vi "PicoScope6000GetTriggerInfo.vi"(0 "handle in":i16, 5 "Segment Range":T1={"fromSegmentIndex"=0, "toSegmentIndex"=9} {"toSegmentIndex" format="%.4p"; "fromSegmentIndex" format="%.4p"}, 9 "Sample Rate":sgl, 11 "error in":errorcluster) -> (4 "handle out":i16, 6 "Trigger Info":T2(array[cluster]), 10 "Trigger Offsets":cluster{u64, sgl}[](array[cluster]) {"?" format="%#_5p"}, 15 "error out":errorcluster)   [LabVIEW 2010]
doc: "This VI gets trigger timestamped data using rapid block mode. It outputs one-dimensional array for each memory segment."
uses:
  ps6000.dll
  shared/Segment Range.ctl
panel:
  out "Number of Captures":u32=1
  in  "fromSegmentIndex":u32
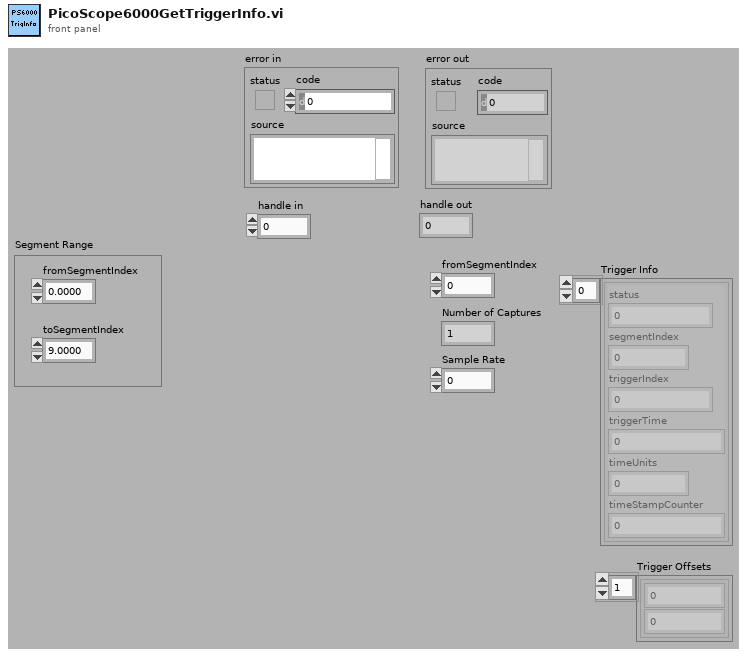
[diagram p1: front panel]
types:
  T1 = typedef "Segment Range.ctl" = cluster{"fromSegmentIndex":u64, "toSegmentIndex":u64}
  T2 = cluster{"status":u32, "segmentIndex":u32, "triggerIndex":u32, "triggerTime":i64, "timeUnits":i16, "timeStampCounter":u64}[]
  T3 = cluster{"status":u32, "segmentIndex":u32, "triggerIndex":u32, "triggerTime":i64, "timeUnits":i16, "reserved0":i16, "timeStampCounter":u64}
  T4 = cluster{"status":bool, "code":u32, "source":string}
  T5 = cluster{"status":u32, "segmentIndex":u32, "triggerIndex":u32, "triggerTime":i64, "timeUnits":i16, "timeStampCounter":u64}
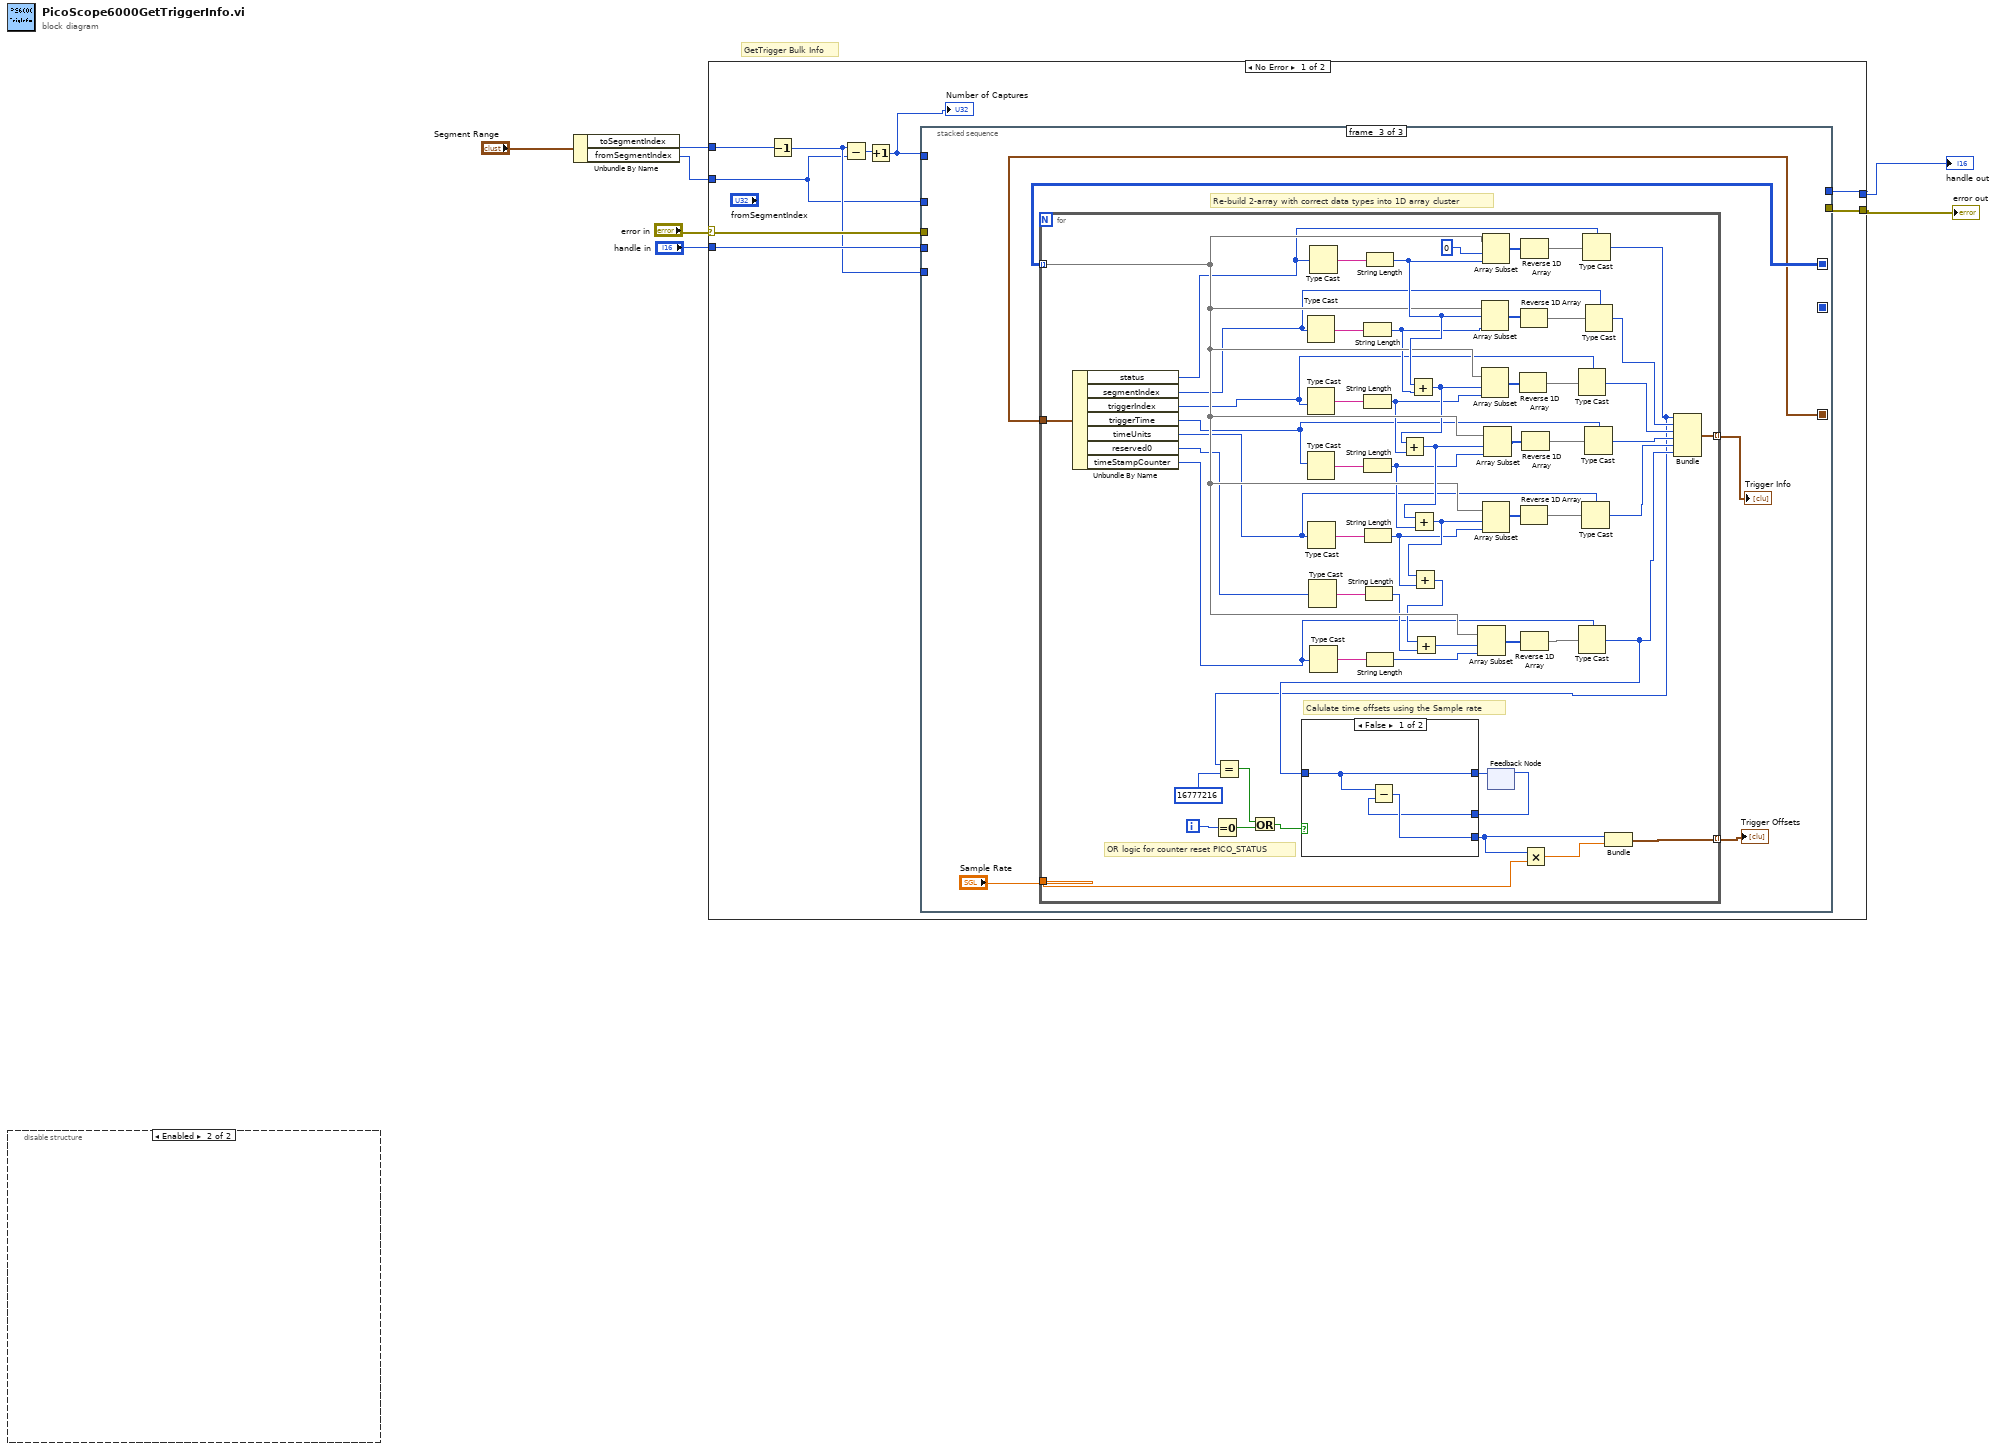
[diagram p0: block diagram]
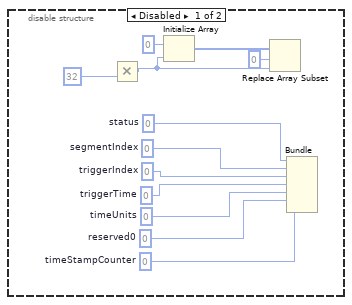
[diagram p2: hidden frame]
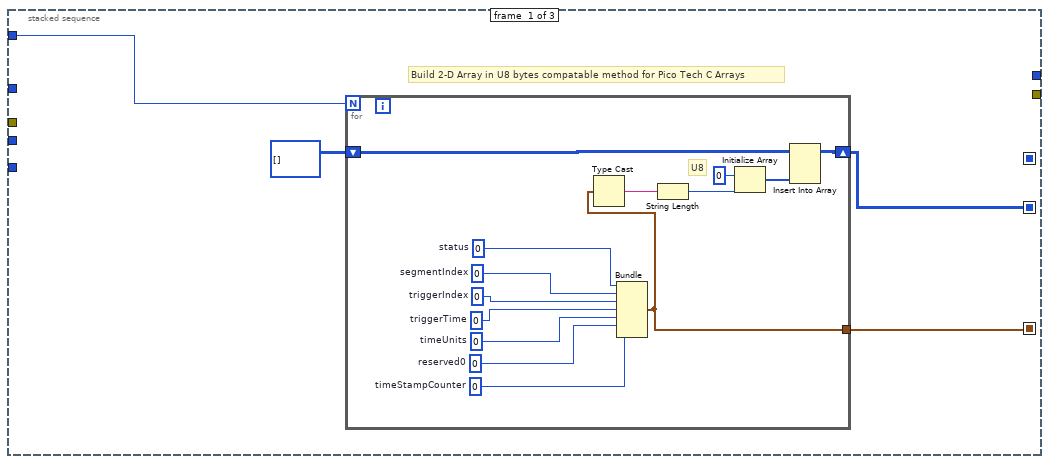
[diagram p3: hidden frame]
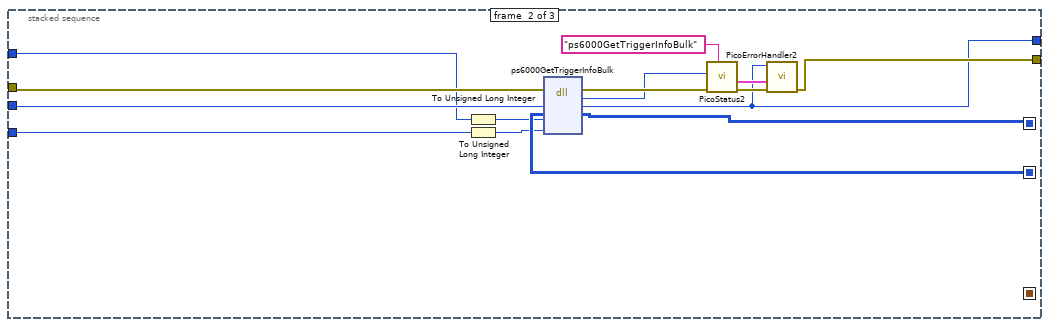
[diagram p4: hidden frame]
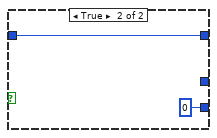
[diagram p5: hidden frame]
diagram:
  # "GetTrigger Bulk Info"
  n1 = disable-structure shown="Enabled" {
    frame Disabled {
      w15 = u64 0  # timeStampCounter
      w13 = i16 0  # reserved0
      w14 = i16 0  # timeUnits
      w16 = i64 0  # triggerTime
      w17 = u32 0  # triggerIndex
      w18 = u32 0  # segmentIndex
      w19 = u32 0  # status
      n2 = Multiply(y=u32 32) -> (x*y=w11:u32)  [unwired: 1 in]
      n3 = Initialize Array(u8 0 ("element"), w11) -> (w12:u8[])
      n4 = Replace Array Subset(array=w12, new element=w11, index=0) -> ()  [unwired: 1 out]
      n5 = Bundle("status"=w19, "segmentIndex"=w18, "triggerIndex"=w17, "triggerTime"=w16, "timeUnits"=w14, "reserved0"=w13, "timeStampCounter"=w15) -> ()  [unwired: 1 in, 1 out]
    }
    frame Enabled {
    }
  }
  n6 = Unbundle By Name("Segment Range") -> ("toSegmentIndex"=w5:u64, "fromSegmentIndex"=w1:u64)
  n7 = case shown="No Error" "error in" {
    selector: "error in" -> [w28 w133]
    tunnel: [w25 w133] -> w3
    tunnel: "handle in" -> [w27 w132]
    tunnel: [w24 w132] -> w4
    tunnel: w5 -> [w21 _]
    tunnel: w1 -> [w22 _]
    frame No Error {
      n8 = Decrement(x=w21) -> (x-1=w26:u64)
      n9 = Subtract(x=w26, y=w22) -> (x-y=w23:u64)
      n10 = Increment(x=w23) -> (x+1=w20:u64)
      "Number of Captures" <- w20
      n11 = stacked-sequence {
        seq-local: [w30 _ _] -> [_ w60 _]
        seq-local: [w29 _ _] -> [_ w58 _]
        seq-local: [_ w59 _] -> [_ _ w67]
        seq-local: [_ w58 _] -> [_ _ w63]
        tunnel: w20 -> [w32 _ _]
        tunnel: w28 -> [_ w62 _]
        tunnel: w27 -> [_ w61 _]
        tunnel: w22 -> [_ w49 _]
        tunnel: w26 -> [_ w48 _]
        tunnel: [_ w55 _] -> w25
        tunnel: [_ w51 _] -> w24
        frame #0 {
          # "Build 2-D Array in U8 bytes compatable method for Pico Tech C Arrays"
          n12 = for {
            N: w32 -> [_]
            shift-right: [w34] -> w30
            shift-left: u8[][] [] -> [w35]
            tunnel: [w33] -> w29
            w42 = u64 0  # timeStampCounter
            w40 = i16 0  # reserved0
            w41 = i16 0  # timeUnits
            w43 = i64 0  # triggerTime
            w44 = u32 0  # triggerIndex
            w45 = u32 0  # segmentIndex
            w46 = u32 0  # status
            # "U8"
            n13 = Bundle("status"=w46, "segmentIndex"=w45, "triggerIndex"=w44, "triggerTime"=w43, "timeUnits"=w41, "reserved0"=w40, "timeStampCounter"=w42) -> (w33:T3)  [unwired: 1 in]
            n14 = Type Cast(x=w33) -> (*(type *) &x=w39:string)  [unwired: 1 in]
            n15 = String Length(string=w39) -> (length=w37:i32)
            n16 = Initialize Array(u8 0 ("element"), w37) -> (w36:u8[])
            n17 = Insert Into Array(array=w35, new element=w36) -> (w34:u8[][])  [unwired: 2 in]
          }
        }
        frame #1 {
          n18 = To Unsigned Long Integer(number=w49) -> (unsigned 32bit integer=w50:u32)
          n19 = To Unsigned Long Integer(number=w48) -> (unsigned 32bit integer=w47:u32)
          n20 = dll-call lib="ps6000.dll" fn="ps6000GetTriggerInfoBulk" ("ps3000.dll:_ps3000_open_unit@0")(error in=w62, "handle"=w61, "triggerInfo"=w60, "fromSegmentIndex"=w50, "toSegmentIndex"=w47) -> (error out=w57:errorcluster, "PICO_STATUS"=w52:u32, "handle"=w51:i16, "triggerInfo"=w59:u8[][])  [unwired: 4 in, 1 out]
          n21 = call "PicoStatus2.vi"("PICO source"="ps6000GetTriggerInfoBulk" ("source"), "Error in"=w57, "PICO STATUS"=w52) -> ("error out"=w56:errorcluster, "PICO_STATUS out"=w54:T4)  [unwired: 5 in]
          n22 = call "PicoErrorHandler2.vi"("error in (no error)"=w56, "PICO_STATUS in"=w54, "handle In"=w51) -> ("error out"=w55:errorcluster)  [unwired: 8 in]
        }
        frame #2 {
          # "Re-build 2-array with correct data types into 1D array cluster"
          n23 = for {
            tunnel: w67 -> [w88] mode=indexing
            tunnel: [w123] -> w66 mode=indexing
            tunnel: [w106] -> w65 mode=indexing
            tunnel: "Sample Rate" -> [w105]
            tunnel: w63 -> [w75]
            i -> [w109]
            # "Calulate time offsets using the Sample rate"
            # "OR logic for counter reset PICO_STATUS"
            n24 = Unbundle By Name(w75) -> ("status"=w74:u32, "segmentIndex"=w73:u32, "triggerIndex"=w68:u32, "triggerTime"=w69:i64, "timeUnits"=w70:i16, "reserved0"=w71:i16, "timeStampCounter"=w72:u64)
            n25 = Equal To 0?(x=w109) -> (x = 0?=w80:bool)
            n26 = Type Cast(x=w73) -> (*(type *) &x=w101:string)  [unwired: 1 in]
            n27 = Type Cast(x=w68) -> (*(type *) &x=w100:string)  [unwired: 1 in]
            n28 = Type Cast(x=w69) -> (*(type *) &x=w99:string)  [unwired: 1 in]
            n29 = Type Cast(x=w70) -> (*(type *) &x=w98:string)  [unwired: 1 in]
            n30 = Type Cast(x=w71) -> (*(type *) &x=w97:string)  [unwired: 1 in]
            n31 = Type Cast(x=w74) -> (*(type *) &x=w102:string)  [unwired: 1 in]
            n32 = Type Cast(x=w72) -> (*(type *) &x=w92:string)  [unwired: 1 in]
            n33 = String Length(string=w101) -> (length=w86:i32)
            n34 = String Length(string=w100) -> (length=w84:i32)
            n35 = String Length(string=w99) -> (length=w83:i32)
            n36 = String Length(string=w98) -> (length=w82:i32)
            n37 = String Length(string=w97) -> (length=w81:i32)
            n38 = String Length(string=w102) -> (length=w93:i32)
            n39 = String Length(string=w92) -> (length=w90:i32)
            n40 = Add(x=w93, y=w86) -> (x+y=w85:i32)
            n41 = Add(x=w85, y=w84) -> (x+y=w96:i32)
            n42 = Add(x=w96, y=w83) -> (x+y=w95:i32)
            n43 = Add(x=w95, y=w82) -> (x+y=w87:i32)
            n44 = Add(x=w87, y=w81) -> (x+y=w91:i32)
            n45 = Array Subset(array=w88, index=w91, length=w90) -> (w89:u8[])
            n46 = Array Subset(array=w88, index=w93, length=w86) -> (w122:u8[])
            n47 = Array Subset(array=w88, index=w85, length=w84) -> (w117:u8[])
            n48 = Array Subset(array=w88, index=0, length=w93) -> (w120:u8[])
            n49 = Array Subset(array=w88, index=w95, length=w82) -> (w114:u8[])
            n50 = Array Subset(array=w88, index=w96, length=w83) -> (w116:u8[])
            n51 = feedback #1() -> (w107:u64)  [unwired: 1 in]
            n52 = Reverse 1D Array(array=w117) -> (reversed array=w118:u8[])
            n53 = Reverse 1D Array(array=w122) -> (reversed array=w121:u8[])
            n54 = Reverse 1D Array(array=w114) -> (reversed array=w113:u8[])
            n55 = Reverse 1D Array(array=w120) -> (reversed array=w119:u8[])
            n56 = Reverse 1D Array(array=w89) -> (reversed array=w112:u8[])
            n57 = Reverse 1D Array(array=w116) -> (reversed array=w115:u8[])
            n58 = Type Cast(type=w68, x=w118) -> (*(type *) &x=w126:u32)
            n59 = Type Cast(type=w72, x=w112) -> (*(type *) &x=w110:u64)
            n60 = Type Cast(type=w70, x=w113) -> (*(type *) &x=w124:i16)
            n61 = Type Cast(type=w74, x=w119) -> (*(type *) &x=w76:u32)
            n62 = Equal?(x=w76, y=u32 16777216 ("status")) -> (x = y?=w78:bool)
            n63 = Or(x=w78, y=w80) -> (x .or. y?=w79:bool)
            n64 = case shown="False" w79 {
              tunnel: w110 -> [w128 w131]
              tunnel: [w128 w131] -> w108
              tunnel: w107 -> [w127 _]
              tunnel: [w129 u64 0] -> w104
              frame False {
                n65 = Subtract(x=w128, y=w127) -> (x-y=w129:u64)
              }
              frame True {
              }
            }
            n66 = feedback-in #1(w108) -> ()
            n67 = Multiply(x=w104, y=w105) -> (x*y=w103:sgl)
            n68 = Type Cast(type=w69, x=w115) -> (*(type *) &x=w125:i64)
            n69 = Type Cast(type=w73, x=w121) -> (*(type *) &x=w111:u32)
            n70 = Bundle(w104, w103) -> (w106:cluster{u64, sgl})  [unwired: 1 in]
            n71 = Bundle("status"=w76, "segmentIndex"=w111, "triggerIndex"=w126, "triggerTime"=w125, "timeUnits"=w124, "timeStampCounter"=w110) -> (w123:T5)  [unwired: 1 in]
          }
          "Trigger Info" <- w66
          "Trigger Offsets" <- w65
        }
      }
    }
    frame Error {
    }
  }
  "handle out" <- w4
  "error out" <- w3
